vi "Write ITX (XY2).vi"(4 "Commands":string, 6 "Notes":string, 8 "error in":errorcluster, 9 "Wavenames":string[](array[string]), 10 "array of clusters":cluster{"Y  Array":dbl[]}[](array[cluster]), 11 "filename":path) -> (0 "error out":errorcluster, 3 "file":path)   [LabVIEW 2019, in "LV-Data.ITX.lvclass"]
uses:
  LV-Data.ITX.lvclass
panel:
  out "String":string
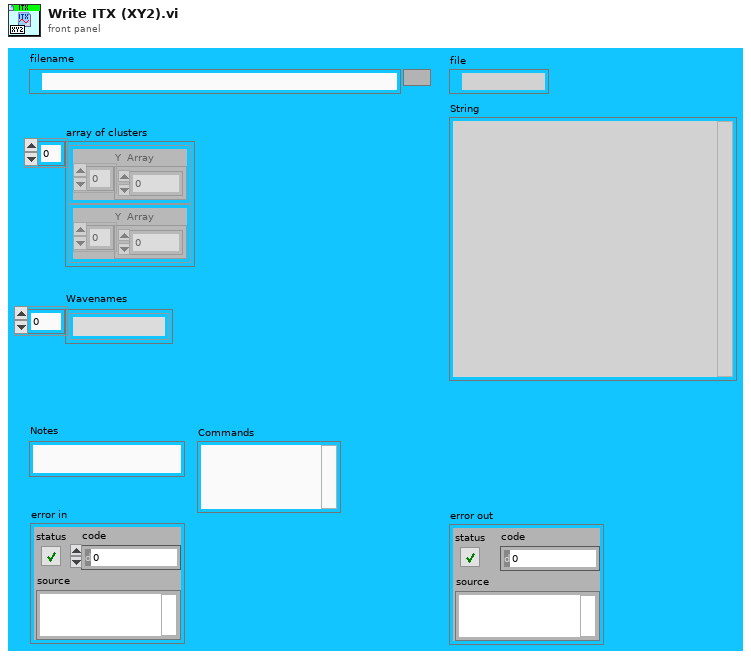
[diagram p1: front panel]
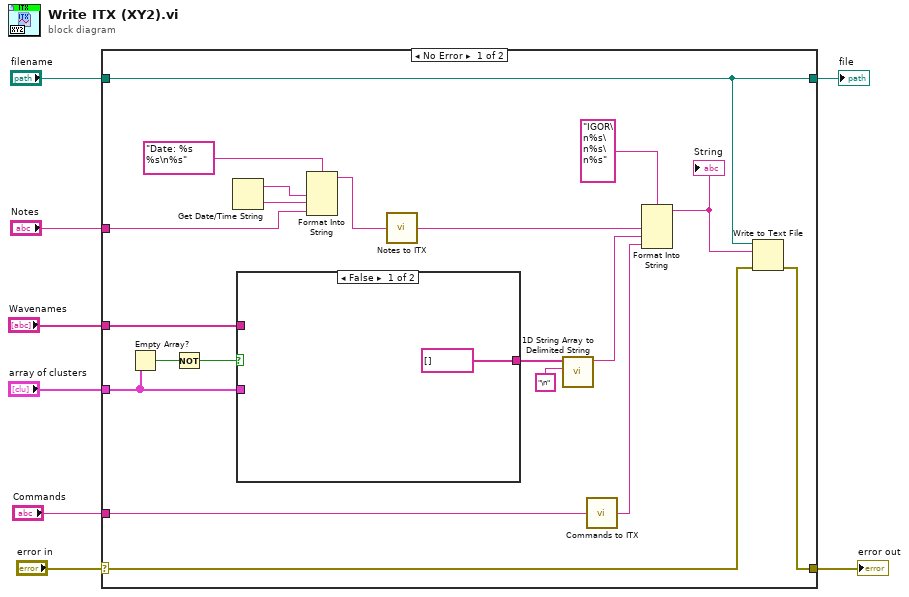
[diagram p0: block diagram]
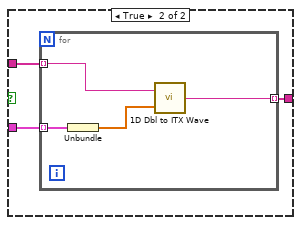
[diagram p2: hidden frame]
diagram:
  n1 = case shown="No Error" "error in" {
    selector: "error in" -> [w24 w38]
    tunnel: "Notes" -> [w16 _]
    tunnel: "array of clusters" -> [w23 _]
    tunnel: "filename" -> [w25 w37]
    tunnel: [w27 w38] -> w5
    tunnel: [w25 w37] -> w4
    tunnel: "Wavenames" -> [w22 _]
    tunnel: "Commands" -> [w21 _]
    frame No Error {
      n2 = Empty Array?(array=w23) -> (empty?=w28:bool)
      n3 = Not(x=w28) -> (.not. x?=w26:bool)
      n4 = Get Date/Time String() -> (date string=w19:string, time string=w18:string)  [unwired: 3 out]
      n5 = case shown="False" w26 {
        tunnel: w23 -> [_ w32]
        tunnel: w22 -> [_ w31]
        tunnel: [string[] [] w30] -> w12
        frame False {
        }
        frame True {
          n6 = for {
            tunnel: w32 -> [w36] mode=indexing
            tunnel: w31 -> [w34] mode=indexing
            tunnel: [w33] -> w30 mode=indexing
            n7 = Unbundle(w36) -> ("Y  Array"=w35:dbl[])
            n8 = call "1D Dbl to ITX Wave.vi"("1D Array"=w35, "Wavename"=w34) -> ("ITX Wave"=w33:string)
          }
        }
      }
      n9 = Format Into String(format string="Date: %s %s\n%s", w19, w18, w16) -> (resulting string=w17:string)  [unwired: 2 in, 1 out]
      n10 = call "Notes to ITX.vi"("Notes"=w17) -> ("ITX Notes"=w14:string)
      n11 = call <vilib>:"1D String Array to Delimited String.vi"("delimiter"="\n" ("delimiter (Tab)"), "string array"=w12) -> ("delimited string"=w10:string)  [unwired: 9 in]
      n12 = call "Commands to ITX.vi"("Commands"=w21) -> ("ITX Commands"=w9:string)
      n13 = Format Into String(format string="IGOR\n%s\n%s\n%s", w14, w10, w9) -> (resulting string=w11:string)  [unwired: 2 in, 1 out]
      "String" <- w11
      n14 = Write to Text File(file (use dialog)=w25, text=w11, error in=w24) -> (error out=w27:errorcluster)  [unwired: 3 out]
    }
    frame Error {
    }
  }
  "file" <- w4
  "error out" <- w5
